vi "B.3.загрузка корневого каталога.vi"(11 "path":string) -> (0 "error out":errorcluster)   [LabVIEW 2011]
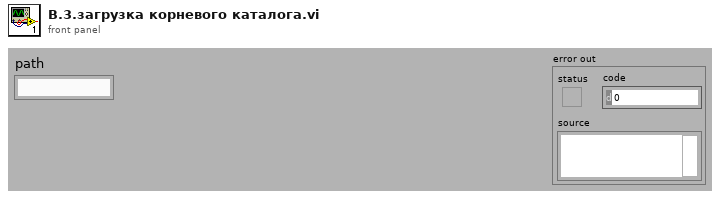
[diagram p1: front panel]
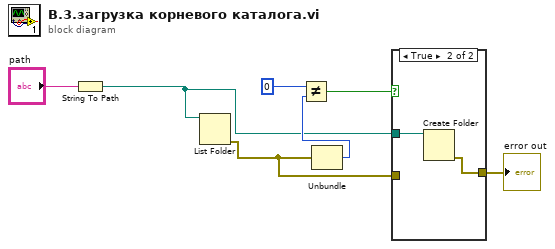
[diagram p0: block diagram]
diagram:
  n1 = String To Path(string="path") -> (path=w2:path)
  n2 = List Folder(path=w2) -> (error out=w4:errorcluster)  [unwired: 3 in, 3 out]
  n3 = Unbundle(w4) -> ("code"=w7:i32)  [unwired: 2 out]
  n4 = Not Equal?(x=0, y=w7) -> (x != y?=w5:bool)
  n5 = case shown="True" w5 {
    tunnel: w2 -> [_ w10]
    tunnel: [w8 w9] -> w3
    tunnel: w4 -> [w8 _]
    frame False {
    }
    frame True {
      n6 = Create Folder(path (use dialog)=w10) -> (error out=w9:errorcluster)  [unwired: 2 in, 2 out]
    }
  }
  "error out" <- w3
